vi "ramps_gen.vi"(0 "Amp":fxp<+/-,20,5>=1.0, 1 "Delay time 10us":i32=1, 5 "error in (no error)":errorcluster, 6 "Ramp1 time 10us":i32=1000, 8 "Ramp2 time 10us":i32=2000, 10 "Ramp3 time 10us":i32=1000, 12 "End time 10us":i32=1) -> (14 "End Address":u32, 19 "error out":errorcluster)   [LabVIEW 2024]
uses:
  <vilib>/rvi/Emulation/niFpgaSctlEmulationGetInTimedLoop.vi
  <vilib>/rvi/Emulation/niFpgaProcessEmulError.vi
  <vilib>/rvi/Memory/Memory_Emulation/nirvimemoryEmulation.vi
  <vilib>/rvi/Memory/Memory_Emulation/nirvimemoryFastEmulation.vi
  <vilib>/rvi/DataTransferAndStorage/Container/Common/niFpgaContainerGetUniqueNameForEmu.vi
  <vilib>/rvi/Memory/Memory_Emulation/niFpgaMemoryEmulationCacheClearOnFirstRun.vi
  <vilib>/rvi/Memory/Memory_Emulation/nirvimemoryEmulationManagerCache_MakeExclusive.vi
  <vilib>/rvi/Memory/Memory_Emulation/niFpgaMemoryEmulationValidateCache.vi
  <vilib>/rvi/Memory/Memory_Emulation/nirvimemoryEmulationManagerCache_InsertValue.vi
  <vilib>/Utility/error.llb/Clear Errors.vi
  <vilib>/rvi/Memory/Memory_Emulation/nirvimemoryEmulationManagerCache_ReleaseExclusive.vi
  <vilib>/rvi/Memory/Memory_Emulation/nirvimemoryEmulationManagerCache_GetValue.vi
  <vilib>/rvi/Emulation/niFpgaEmulationIsFPGAContextNoSignature.vi
  <vilib>/rvi/Memory/Memory_Emulation/nirvimemoryEmulationManagerCache_SetValue.vi
  <vilib>/rvi/Emulation/niFpgaSctlEmulationResourceMgr.vi
  <vilib>/rvi/DataTransferAndStorage/Container/XNode/niFpgaContainer.xnode
panel:
  # "Time should be in unit of 10us, assuming 100kHz frequency"
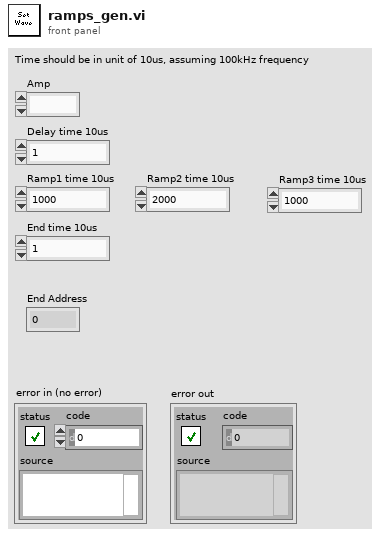
[diagram p1: front panel]
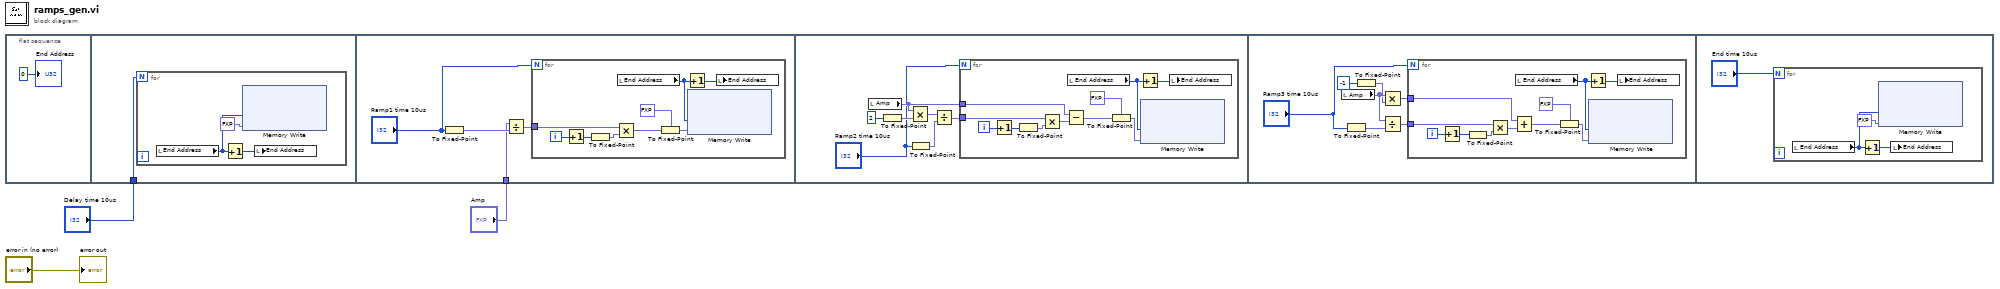
[diagram p0: block diagram]
diagram:
  n1 = flat-sequence {
    tunnel: "Delay time 10us" -> [w5]
    tunnel: "Amp" -> [w10]
    frame #0 {
      "End Address" <- u32 0 ("End Address")
    }
    frame #1 {
      n2 = for {
        N: w5 -> [_]
        n3 = local read "End Address"() -> (w7:u32)
        n4 = Increment(x=w7) -> (x+1=w8:u32)
        n5 = xnode ("Memory Write")("Address"=w7, "Data"=fxp<+/-,20,5> 0.0) -> ()  [unwired: 1 in, 1 out]
        n6 = local write "End Address"(w8) -> ()
      }
    }
    frame #2 {
      n7 = To Fixed-Point(number="Ramp1 time 10us") -> (fixed-point=w11:fxp<+/-,32,32>)  [unwired: 1 in]
      n8 = Divide(x=w10, y=w11) -> (x/y=w9:fxp<+/-,32,6>)
      n9 = for {
        N: "Ramp1 time 10us" -> [_]
        tunnel: w9 -> [w21]
        i -> [w20]
        n10 = Increment(x=w20) -> (x+1=w15:i32)
        n11 = To Fixed-Point(number=w15) -> (fixed-point=w14:fxp<+/-,32,32>)  [unwired: 1 in]
        n12 = Multiply(x=w21, y=w14) -> (x*y=w19:fxp<+/-,64,38>)
        n13 = local read "End Address"() -> (w17:u32)
        n14 = To Fixed-Point(fixed-point type=fxp<+/-,20,5> 0.0, number=w19) -> (fixed-point=w18:fxp<+/-,20,5>)
        n15 = Increment(x=w17) -> (x+1=w16:u32)
        n16 = xnode ("Memory Write")("Address"=w17, "Data"=w18) -> ()  [unwired: 1 in, 1 out]
        n17 = local write "End Address"(w16) -> ()
      }
    }
    frame #3 {
      n18 = local read "Amp"() -> (w28:fxp<+/-,20,5>)
      n19 = To Fixed-Point(number=i16 2 ("y")) -> (fixed-point=w26:fxp<+/-,16,16>)  [unwired: 1 in]
      n20 = Multiply(x=w28, y=w26) -> (x*y=w25:fxp<+/-,36,21>)
      n21 = To Fixed-Point(number="Ramp2 time 10us") -> (fixed-point=w24:fxp<+/-,32,32>)  [unwired: 1 in]
      n22 = Divide(x=w25, y=w24) -> (x/y=w23:fxp<+/-,32,6>)
      n23 = for {
        N: "Ramp2 time 10us" -> [_]
        tunnel: w28 -> [w39]
        tunnel: w23 -> [w36]
        i -> [w35]
        n24 = Increment(x=w35) -> (x+1=w38:i32)
        n25 = To Fixed-Point(number=w38) -> (fixed-point=w29:fxp<+/-,32,32>)  [unwired: 1 in]
        n26 = Multiply(x=w36, y=w29) -> (x*y=w37:fxp<+/-,64,38>)
        n27 = Subtract(x=w39, y=w37) -> (x-y=w31:fxp<+/-,64,38>)
        n28 = local read "End Address"() -> (w34:u32)
        n29 = To Fixed-Point(fixed-point type=fxp<+/-,20,5> 0.0 ("Data"), number=w31) -> (fixed-point=w30:fxp<+/-,20,5>)
        n30 = Increment(x=w34) -> (x+1=w33:u32)
        n31 = xnode ("Memory Write")("Address"=w34, "Data"=w30) -> ()  [unwired: 1 in, 1 out]
        n32 = local write "End Address"(w33) -> ()
      }
    }
    frame #4 {
      n33 = local read "Amp"() -> (w44:fxp<+/-,20,5>)
      n34 = To Fixed-Point(number="Ramp3 time 10us") -> (fixed-point=w42:fxp<+/-,32,32>)  [unwired: 1 in]
      n35 = To Fixed-Point(number=i16 -1 ("y")) -> (fixed-point=w43:fxp<+/-,16,16>)  [unwired: 1 in]
      n36 = Multiply(x=w44, y=w43) -> (x*y=w45:fxp<+/-,36,21>)
      n37 = Divide(x=w44, y=w42) -> (x/y=w41:fxp<+/-,53,6>)
      n38 = for {
        N: "Ramp3 time 10us" -> [_]
        tunnel: w45 -> [w57]
        tunnel: w41 -> [w56]
        i -> [w54]
        n39 = Increment(x=w54) -> (x+1=w48:i32)
        n40 = To Fixed-Point(number=w48) -> (fixed-point=w47:fxp<+/-,32,32>)  [unwired: 1 in]
        n41 = Multiply(x=w56, y=w47) -> (x*y=w55:fxp<+/-,32,6>)
        n42 = Add(x=w57, y=w55) -> (x+y=w49:fxp<+/-,47,21>)
        n43 = local read "End Address"() -> (w53:u32)
        n44 = To Fixed-Point(fixed-point type=fxp<+/-,20,5> 0.0 ("Data"), number=w49) -> (fixed-point=w50:fxp<+/-,20,5>)
        n45 = Increment(x=w53) -> (x+1=w52:u32)
        n46 = xnode ("Memory Write")("Address"=w53, "Data"=w50) -> ()  [unwired: 1 in, 1 out]
        n47 = local write "End Address"(w52) -> ()
      }
    }
    frame #5 {
      n48 = for {
        N: "End time 10us" -> [_]
        n49 = local read "End Address"() -> (w61:u32)
        n50 = Increment(x=w61) -> (x+1=w59:u32)
        n51 = xnode ("Memory Write")("Address"=w61, "Data"=fxp<+/-,20,5> 0.0) -> ()  [unwired: 1 in, 1 out]
        n52 = local write "End Address"(w59) -> ()
      }
    }
  }
  "error out" <- "error in (no error)"
